vi "SVPO Limit Testing (N Ch) (SGL Array).vi"(7 "reset? (F)":bool, 9 "lower limit":sgl=-inf format="%.2f", 10 "upper limit":sgl=inf format="%.2f", 11 "signals in":sgl[][](array[numeric])) -> (1 "lower limit clearances":sgl[](array[numeric]) format="%.6f", 2 "upper limit clearances":sgl[](array[numeric]) format="%.6f", 3 "tests passed?":bool[](array[boolean]))   [LabVIEW 2017, in "SoundVib_LimitTest.lvlib"]
doc: "Performs limit testing on single-precision waveforms, single-precision scaled arrays, or double-precision scalar measurements. You can specify an upper and lower boundary of the envelope to define a pass range. This VI uses the defined pass range to test the input signal. VI outputs apply to all the tests since the last VI reset. Use this VI on embedded targets that have limited computational resources. Wire data to the <B>value in</B> input to determine the polymorphic instance to use or manually select the instance."
uses:
  <vilib>/addons/Sound and Vibration/svt_Limit Test/SoundVib_LimitTest.lvlib
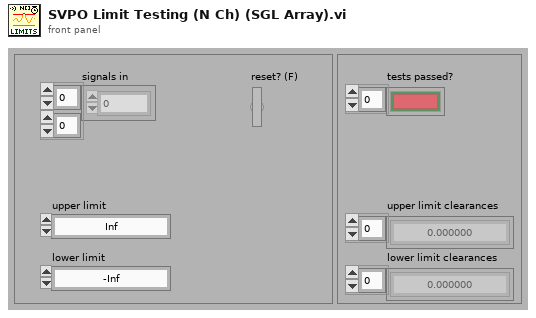
[diagram p1: front panel]
types:
  T1 = typedef "svc_SGL Limit State.ctl" = cluster{"upper limit clearance":sgl, "lower limit clearance":sgl, "test passed?":bool, "block passed?":bool}
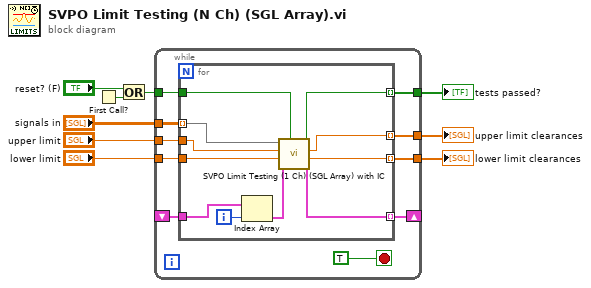
[diagram p0: block diagram]
diagram:
  n1 = First Call?() -> (First Call?: T/F=w6:bool)
  n2 = Or(x="reset? (F)", y=w6) -> (x .or. y?=w7:bool)
  n3 = while {
    tunnel: "signals in" -> [w19]
    tunnel: "upper limit" -> [w17]
    tunnel: "lower limit" -> [w15]
    tunnel: w7 -> [w18]
    shift-right: [w13] -> _
    shift-left: _ -> [w14]
    tunnel: [w12] -> w3
    tunnel: [w11] -> w2
    tunnel: [w10] -> w1
    stop <- TRUE stop-if-true
    n4 = for {
      tunnel: w19 -> [w30] mode=indexing
      tunnel: w18 -> [w23]
      tunnel: w17 -> [w29]
      tunnel: w15 -> [w28]
      tunnel: w14 -> [w25]
      tunnel: [w27] -> w13 mode=indexing
      tunnel: [w22] -> w12 mode=indexing
      tunnel: [w21] -> w11 mode=indexing
      tunnel: [w20] -> w10 mode=indexing
      i -> [w26]
      n5 = Index Array(array=w25, index=w26) -> (element=w24:T1)
      n6 = call <vilib>:"SVPO Limit Testing (1 Ch) (SGL Array) with IC.vi"("reset? (F)"=w23, "initial conditions"=w24, "lower limit"=w28, "upper limit"=w29, "signal in"=w30) -> ("final conditions"=w27:T1, "lower limit clearance"=w20:sgl, "upper limit clearance"=w21:sgl, "test passed?"=w22:bool)  [unwired: 3 in]
    }
  }
  "tests passed?" <- w3
  "upper limit clearances" <- w2
  "lower limit clearances" <- w1
